vi "SAI.vi"(0 "System no.":i32=1 min=1 max=4 step=1, 2 "Old axis ID":string[](array[string]), 3 "New axis ID":string[](array[string]), 5 "error in":errorcluster) -> (19 "error out":errorcluster)   [LabVIEW 2020]
doc: "Set axis identifier. With this command the axis identifiers of the connected axes can be changed. \nGCS 1.0: Only one character is allowed as axis ID. Valid axis IDs can be listed with TVI?.vi. \nGCS 2.0: Characters that Axis IDs can contain can be listet with TVI?.vi. \nPlease run Define connected axes.vi with new axis IDs after renaming axes.\n\nE-517, E-518: Maximum length for axis name is 8 characters. SAI affects the Axis Name parameter, ID 0x07000600, in volatile memory (RAM). To save the currently valid value to non-volatile memory, where it becomes the power-on default, you must use WPA. Changes not saved with WPA will be lost when the controller is powered down or rebooted.\n\nE-709: Maximum length for axis name is 4 characters. SAI affects the Axis Name parameter, ID 0x07000600, in volatile memory (RAM). To save the currently valid value to non-volatile memory, where it becomes the power-on default, you must use WPA. Changes not saved with WPA will be lost when the controller is powered down or rebooted.\n\nC-867, C-877, C-884, C-891, E-761, E-871, E-873, E-874, Mercury_GCS: The settings are automatically written to non-volatile memory.\n\nHydra, Pollux: To save the currently valid axis identifier to non-volatile memory, where it becomes the power-on default, you must use WPA. Changes not saved with WPA will be lost when the controller is powered down or rebooted."
panel:
  # "Set axis identifier. With this command the axis identifiers of the\nconnected axes can be changed. \nGCS 1.0: Only one character is allowed as axis ID. Valid axis IDs can be \nlisted with TVI?.vi. \nGCS 2.0: Characters that Axis IDs can contain can be listet with TVI?.vi. \nPlease run \"Define connected axes.vi\" with new axis IDs after \nrenaming axes."
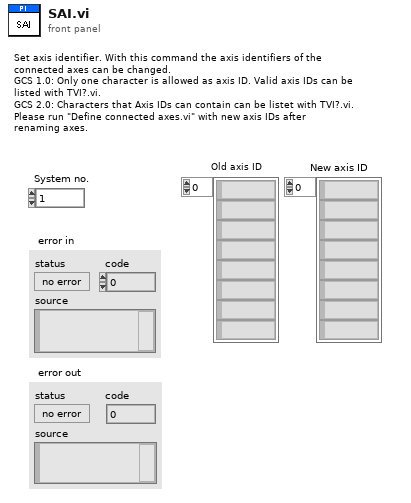
[diagram p1: front panel]
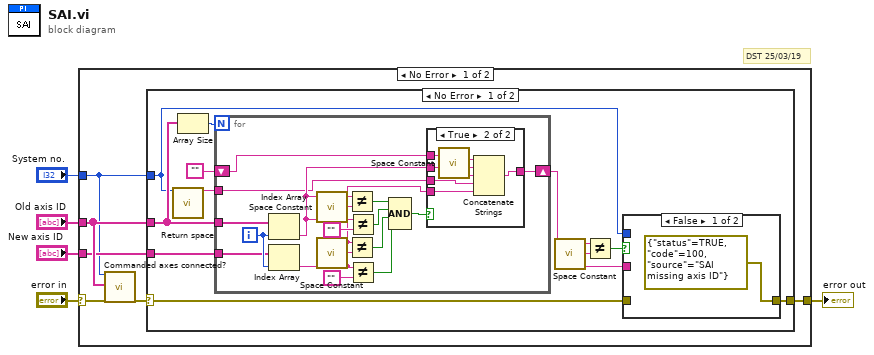
[diagram p0: block diagram]
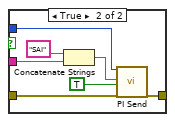
[diagram p2: hidden frame]
diagram:
  # "DST 25/03/19"
  n1 = case shown="No Error" "error in" {
    selector: "error in" -> [w7 w56]
    tunnel: "Old axis ID" -> [w11 _]
    tunnel: [w10 w56] -> w4
    tunnel: "New axis ID" -> [w9 _]
    tunnel: "System no." -> [w8 _]
    frame No Error {
      n2 = call "Commanded axes connected?.vi"("System no."=w8, "Commanded axes"=w11, "error in"=w7) -> ("error out"=w6:errorcluster)  [unwired: 16 out]
      n3 = case shown="No Error" w6 {
        selector: w6 -> [w12 w55]
        tunnel: w11 -> [w22 _]
        tunnel: [w17 w55] -> w10
        tunnel: w9 -> [w19 _]
        tunnel: w8 -> [w13 _]
        frame No Error {
          n4 = call "Return space.vi"("System no."=w13) -> ("String out"=w14:string)  [unwired: 1 in, 17 out]
          n5 = Array Size(array=w22) -> (size(s)=w15:i32)
          n6 = for {
            N: w15 -> [_]
            tunnel: w22 -> [w36]
            shift-right: [w45] -> w18
            shift-left: "" -> [w46]
            tunnel: w19 -> [w34]
            tunnel: w14 -> [w31]
            i -> [w35]
            n7 = Index Array(array=w36, index=w35) -> (element=w44:string)
            n8 = Index Array(array=w34, index=w35) -> (element=w33:string)
            n9 = call <vilib>:"Space Constant.vi"() -> ("String"=w47:string)
            n10 = call <vilib>:"Space Constant.vi"() -> ("String"=w42:string)
            n11 = Not Equal?(x=w44, y=w47) -> (x != y?=w40:bool)
            n12 = Not Equal?(x=w33, y=w42) -> (x != y?=w38:bool)
            n13 = Not Equal?(x=w44, y="") -> (x != y?=w39:bool)
            n14 = Not Equal?(x=w33, y="") -> (x != y?=w37:bool)
            n15 = Compound Arithmetic op=AND(w40, w39, w38, w37) -> (w32:bool)
            n16 = case shown="True" w32 {
              tunnel: w46 -> [w48 w54]
              tunnel: w44 -> [_ w51]
              tunnel: [w48 w53] -> w45
              tunnel: w33 -> [_ w50]
              tunnel: w31 -> [_ w49]
              frame False {
              }
              frame True {
                n17 = call <vilib>:"Space Constant.vi"() -> ("String"=w52:string)
                n18 = Concatenate Strings(w54, w52, w51, w49, w50) -> (w53:string)
              }
            }
          }
          n19 = call <vilib>:"Space Constant.vi"() -> ("String"=w20:string)
          n20 = Not Equal?(x=w18, y=w20) -> (x != y?=w16:bool)
          n21 = case shown="False" w16 {
            tunnel: w18 -> [_ w28]
            tunnel: w12 -> [_ w26]
            tunnel: w13 -> [_ w25]
            tunnel: [errorcluster {"status"=TRUE, "code"=100, "source"="SAI missing axis ID"} ("error out") w24] -> w17
            frame False {
            }
            frame True {
              n22 = Concatenate Strings("SAI", w28) -> (w27:string)
              n23 = call "PI Send.vi"("System no."=w25, "String to send"=w27, "Attach termination char.?"=TRUE ("Attach Linefeed?"), "error in"=w26) -> ("error out"=w24:errorcluster)  [unwired: 2 in, 13 out]
            }
          }
        }
        frame Error {
        }
      }
    }
    frame Error {
    }
  }
  "error out" <- w4
